vi "Global Variables.vi"() -> ()   [LabVIEW 2012]
panel:
  in  "OutPath":path
  in  "Image":T1(plugin-control)
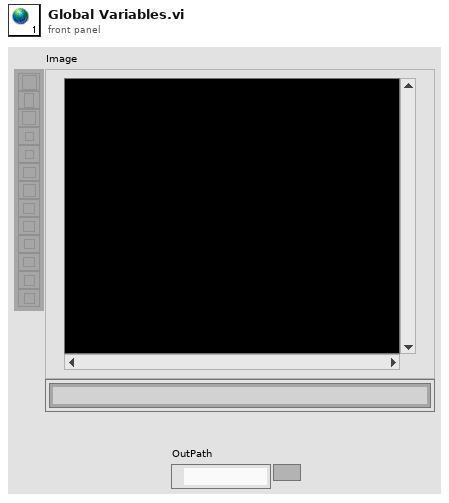
[diagram p1: front panel]
types:
  T1 = typedef "IMAQ Image.ctl" = refnum<image>
diagram:
